vi "浮点数值写入.vi"(7 "浮点":sgl[](array[numeric]), 8 "error in (no error)":errorcluster, 9 "starting address":u16, 10 "Slave ID":u8=1, 11 "MB session in":refnum<class "MB_Master.lvclass">) -> (0 "error out":errorcluster, 3 "MB session out":refnum<class "MB_Master.lvclass">)   [LabVIEW 2016, in "流量计集成.lvlib" / "斯坦道功率测流.lvlib"]
uses:
  <vilib>/Plasmionique/MB Master/MB_Master/MB_Master.lvclass
  <vilib>/Plasmionique/MB Master/MB Master.lvlib
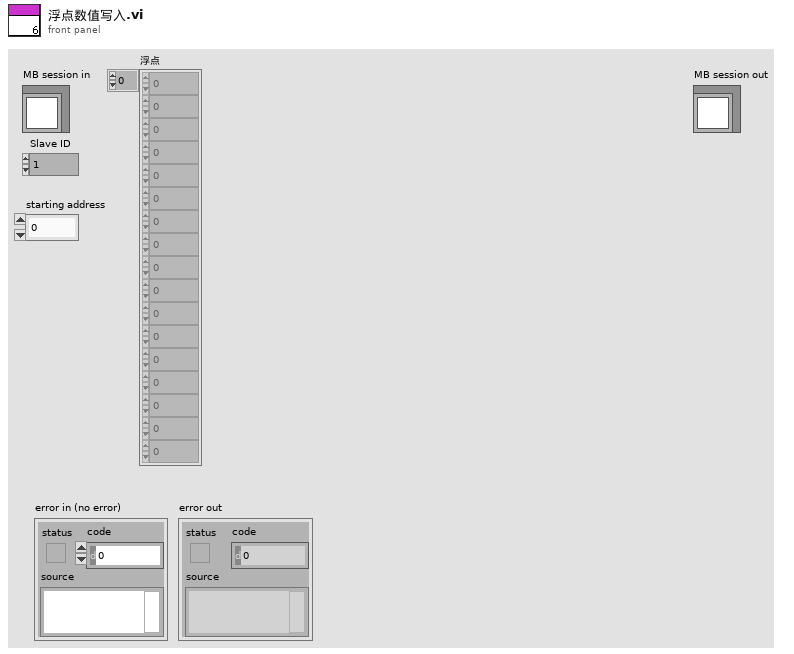
[diagram p1: front panel]
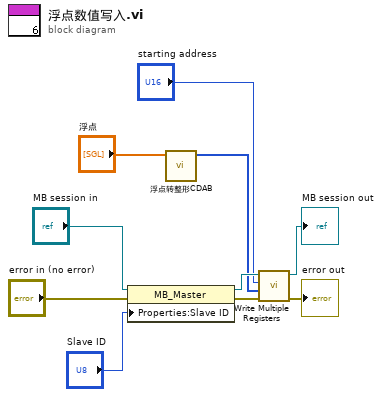
[diagram p0: block diagram]
diagram:
  n1 = property class="MB_Master"(reference="MB session in", error in="error in (no error)", "Properties:Slave ID"="Slave ID") -> (reference out=w7:refnum<class "MB_Master.lvclass">, error out=w5:errorcluster)
  n2 = call "浮点转整形CDAB.vi"("浮点"="浮点") -> ("整形CDAB"=w2:u16[])  [unwired: 10 in]
  n3 = call <vilib>:"Write Multiple Registers.vi"("error in (no error)"=w5, "values"=w2, "starting address"="starting address", "MB session in"=w7) -> ("error out"=→"error out":errorcluster, "MB session out"=→"MB session out":refnum<class "MB_Master.lvclass">)  [unwired: 6 in]
